vi "22.Evd.8_Ask.3.vi"() -> ()   [LabVIEW 2025]
uses:
  <vilib>/Utility/file.llb/Write Delimited Spreadsheet (DBL).vi
panel:
  out "error out":errorcluster
  out "Column Average":dbl
  out "Line Average":dbl
  out "Desired Column":dbl[](array[numeric])
  out "Desired Line":dbl[](array[numeric])
  out "min value":dbl
  out "max value":dbl
  out "Array 2":dbl[][](array[numeric])
  in  "Column Selection":dbl
  in  "Line Selection":dbl
  out "size(s)":i32[](array[numeric])
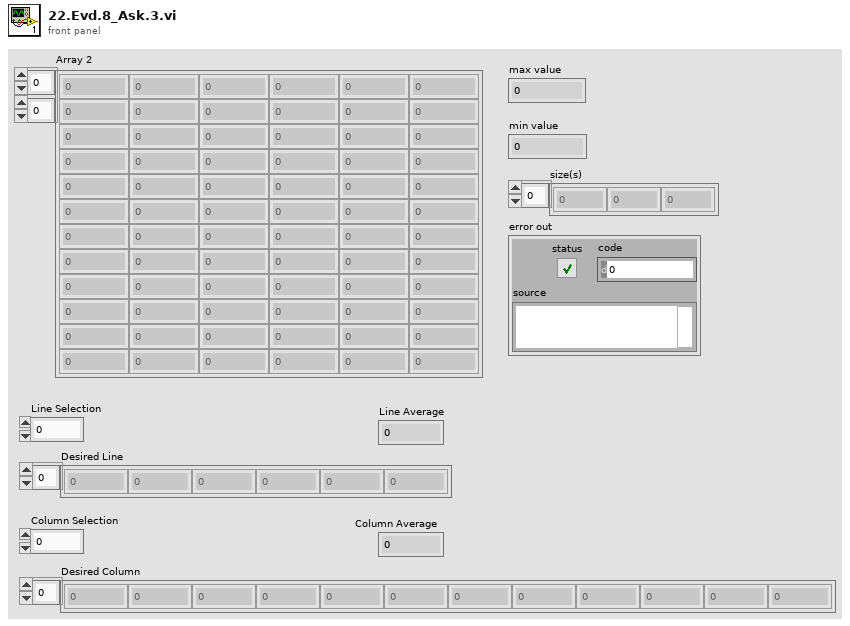
[diagram p1: front panel]
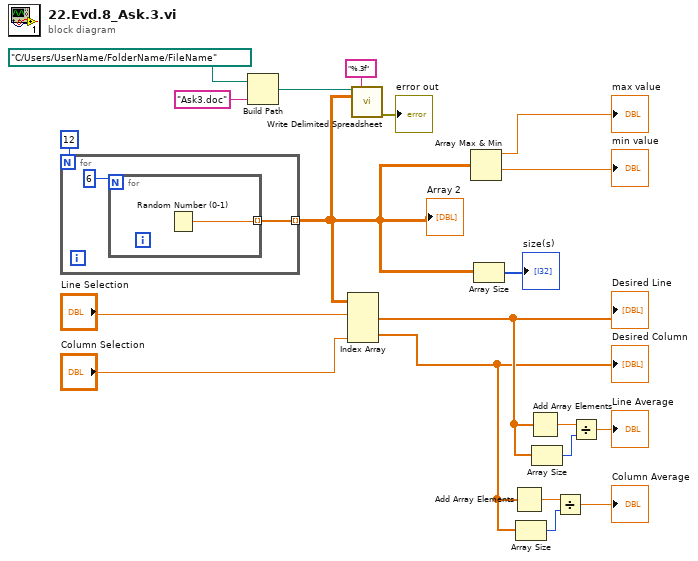
[diagram p0: block diagram]
diagram:
  n1 = for {
    N: 12 -> [_]
    tunnel: [w21] -> w5 mode=indexing
    n2 = for {
      N: 6 -> [_]
      tunnel: [w23] -> w21 mode=indexing
      n3 = Random Number (0-1)() -> (number: 0 to 1=w23:dbl)
    }
  }
  "Array 2" <- w5
  n4 = Build Path(base path=path "C:/Users/UserName/FolderName/FileName", name or relative path="Ask3.doc") -> (appended path=w1:path)
  n5 = Index Array(array=w5, index (row) #1="Line Selection", index (col) #2="Column Selection") -> (element #1=w13:dbl[], element #2=w7:dbl[])  [unwired: 2 in]
  "Desired Line" <- w13
  "Desired Column" <- w7
  n6 = call-poly <vilib>:"Write Delimited Spreadsheet.vi"("file path (dialog if empty)"=w1, "format (%.3f)"="%.3f", "2D data"=w5) -> ("error out"=→"error out":errorcluster)  [unwired: 11 in, 1 out]
  n7 = Array Max & Min(array=w5) -> (max value=→"max value":dbl, min value=→"min value":dbl)  [unwired: 2 out]
  n8 = Array Size(array=w5) -> (size(s)=→"size(s)":i32[])
  n9 = Add Array Elements(numeric array=w7) -> (sum=w10:dbl)
  n10 = Array Size(array=w7) -> (size(s)=w9:i32)
  n11 = Add Array Elements(numeric array=w13) -> (sum=w14:dbl)
  n12 = Array Size(array=w13) -> (size(s)=w12:i32)
  n13 = Divide(x=w10, y=w9) -> (x/y=→"Column Average":dbl)
  n14 = Divide(x=w14, y=w12) -> (x/y=→"Line Average":dbl)
